vi "Graph AddCursor(Wave).vi"(8 "エラー入力（エラーなし）":errorcluster, 9 "色":u32(colorbox), 10 "名称":string, 11 "WaveformGraph入力":refnum<vi>) -> (0 "エラー出力":errorcluster)   [LabVIEW 2014]
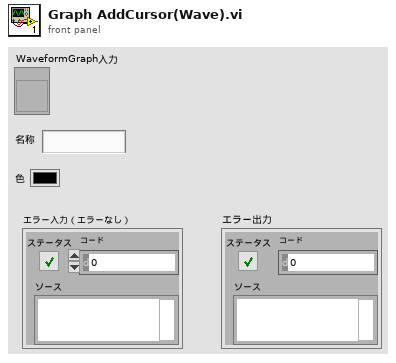
[diagram p1: front panel]
types:
  T1 = cluster{"Name":string, "Color":u32, "Style":u8, "Point Style":u8, "Name Visible":bool, "Allow Drag":bool, "Cursor Mode":u32, "Plot":i32, "Index":i32, "Position":cluster{"X":dbl, "Y":dbl}, "X Scale":u32, "Y Scale":u32, "Watch Plots":i32[], "Watch All Plots":bool, "Plot Area":i32, "Label Offset":cluster{"X":dbl, "Y":dbl}}
  T2 = typedef "LVCursorListTypeDef.ctl" = cluster{"Name":string, "Color":u32, "Style":u8, "Point Style":u8, "Name Visible":bool, "Allow Drag":bool, "Cursor Mode":u32, "Plot":i32, "Index":i32, "Position":cluster{"X":dbl, "Y":dbl}, "X Scale":u32, "Y Scale":u32, "Watch Plots":i32[], "Watch All Plots":bool, "Plot Area":i32, "Label Offset":cluster{"X":dbl, "Y":dbl}}[]
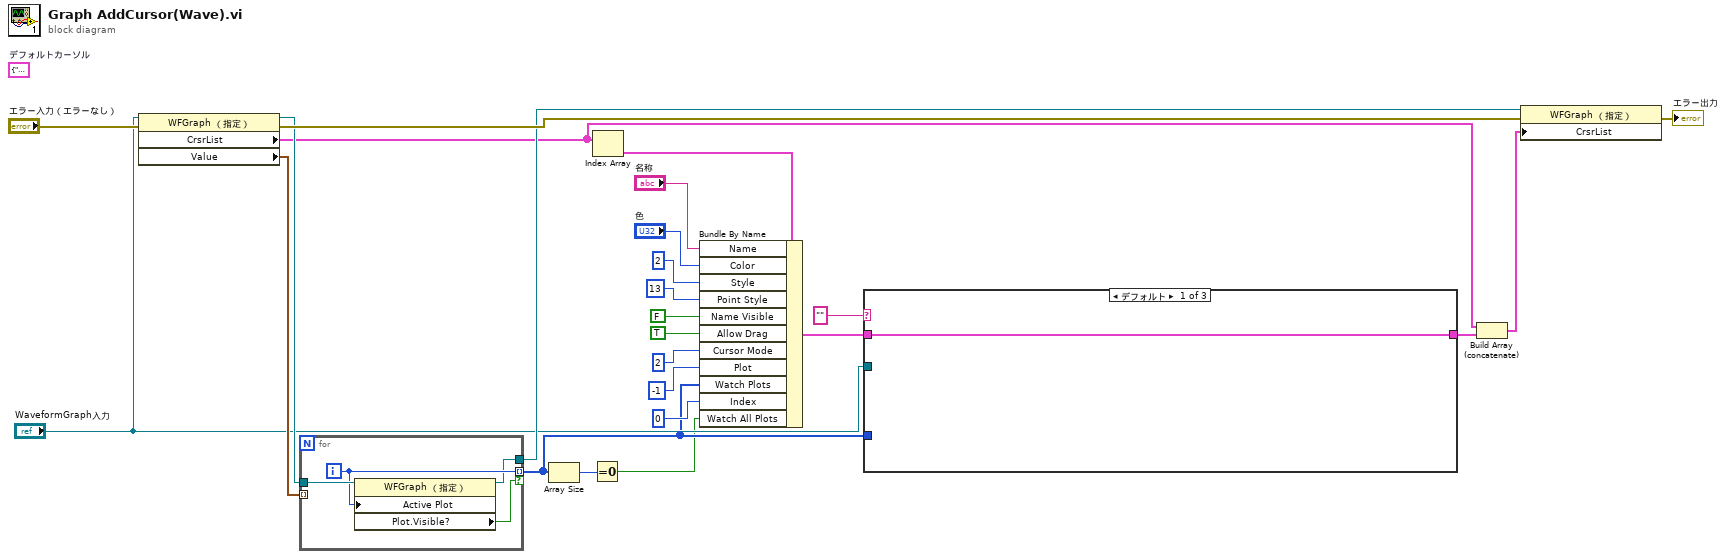
[diagram p0: block diagram]
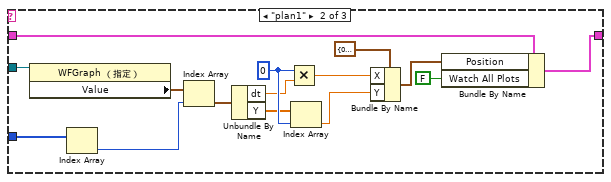
[diagram p2: hidden frame]
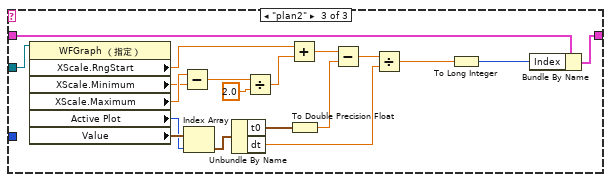
[diagram p3: hidden frame]
diagram:
  (unwired) T1 {"Name"="カーソル0", "Color"=16776960, "Style"=2, "Point Style"=13, "Name Visible"=FALSE, "Allow Drag"=TRUE, "Cursor Mode"=2, "Plot"=-1, "Index"=42, "Position"={"X"=0.42, "Y"=43.0}, "X Scale"=0, "Y Scale"=0, "Watch Plots"=[], "Watch All Plots"=TRUE, "Plot Area"=0, "Label Offset"={"X"=-0.0012080536912751905, "Y"=172.10516252390056}}  # デフォルトカーソル
  n1 = property class="WFGraph （指定）"(reference="WaveformGraph入力", error in="エラー入力（エラーなし）") -> (reference out=w13:refnum<vi>, error out=w19:errorcluster, "CrsrList"=w2:T2, "Value"=w24:waveform(dbl)[])
  n2 = for {
    tunnel: w13 -> [w29]
    tunnel: w24 -> [_] mode=indexing
    tunnel: [w28] -> w10 mode=indexing if=w27
    tunnel: [w26] -> w14
    i -> [w28]
    n3 = property class="WFGraph （指定）"(reference=w29, "Active Plot"=w28) -> (reference out=w26:refnum<vi>, "Plot.Visible?"=w27:bool)  [unwired: 1 in, 1 out]
  }
  n4 = Array Size(array=w10) -> (size(s)=w9:i32)
  n5 = Equal To 0?(x=w9) -> (x = 0?=w8:bool)
  n6 = Index Array(array=w2) -> (element=w1:T1)  [unwired: 1 in]
  n7 = Bundle By Name(cluster=w1, "Name"="名称", "Color"="色", "Style"=u8 2, "Point Style"=u8 13, "Name Visible"=FALSE, "Allow Drag"=TRUE, "Cursor Mode"=u32 2, "Plot"=-1, "Watch Plots"=w10, "Index"=0, "Watch All Plots"=w8) -> (w16:T1)
  n8 = case shown="デフォルト" "" {
    tunnel: w10 -> [_ w45 _]
    tunnel: w16 -> [w30 w33 w62]
    tunnel: [w30 w32 w61] -> w15
    tunnel: "WaveformGraph入力" -> [_ w31 w64]
    frame Default {
    }
    frame "plan1" {
      w43 = 0 ("Index")
      n9 = property class="WFGraph （指定）"(reference=w31) -> ("Value"=w37:waveform(dbl)[])  [unwired: 1 in, 2 out]
      n10 = Index Array(array=w45) -> (element=w38:i32)  [unwired: 1 in]
      n11 = Index Array(array=w37, index=w38) -> (element=w39:waveform(dbl))
      n12 = Unbundle By Name(w39) -> ("dt"=w42:dbl, "Y"=w40:dbl[])
      n13 = Multiply(x=w43, y=w42) -> (x*y=w44:dbl)
      n14 = Index Array(array=w40, index=w43) -> (element=w41:dbl)
      n15 = Bundle By Name(cluster=cluster{"X":dbl, "Y":dbl} {"X"=0.0, "Y"=0.0} ("Position"), "X"=w44, "Y"=w41) -> (w34:cluster{"X":dbl, "Y":dbl})
      n16 = Bundle By Name(cluster=w33, "Position"=w34, "Watch All Plots"=FALSE) -> (w32:T1)
    }
    frame "plan2" {
      n17 = property class="WFGraph （指定）"(reference=w64) -> ("XScale.RngStart"=w56:dbl, "XScale.Minimum"=w59:dbl, "XScale.Maximum"=w60:dbl, "Active Plot"=w54:u32, "Value"=w55:waveform(dbl)[])  [unwired: 1 in, 2 out]
      n18 = Subtract(x=w60, y=w59) -> (x-y=w58:dbl)
      n19 = Index Array(array=w55, index=w54) -> (element=w53:waveform(dbl))
      n20 = Unbundle By Name(w53) -> ("t0"=w49:timestamp, "dt"=w47:dbl)
      n21 = Divide(x=w58, y=2.0) -> (x/y=w57:dbl)
      n22 = Add(x=w56, y=w57) -> (x+y=w51:dbl)
      n23 = To Double Precision Float(number=w49) -> (double precision float=w48:dbl)
      n24 = Subtract(x=w51, y=w48) -> (x-y=w50:dbl)
      n25 = Divide(x=w50, y=w47) -> (x/y=w46:dbl)
      n26 = To Long Integer(number=w46) -> (32bit integer=w52:i32)
      n27 = Bundle By Name(cluster=w62, "Index"=w52) -> (w61:T1)
    }
  }
  n28 = Build Array (concatenate)(w2, w15) -> (w21:T2)
  n29 = property class="WFGraph （指定）"(reference=w14, error in=w19, "CrsrList"=w21) -> (error out=→"エラー出力":errorcluster)  [unwired: 1 out]
